vi "P3060_DMA读U32数据.vi"(8 "错误输入":errorcluster caption="错误输入（无错误）", 9 "数据长度":u32, 10 "偏移地址":u32, 11 "句柄输入":i32) -> (0 "错误输出":errorcluster, 1 "读I64数据":u32[](array[numeric]), 2 "返回值":i32, 3 "句柄输出":i32)   [LabVIEW 2010]
doc: "发送异步通道数据"
uses:
  dll/P3060.dll
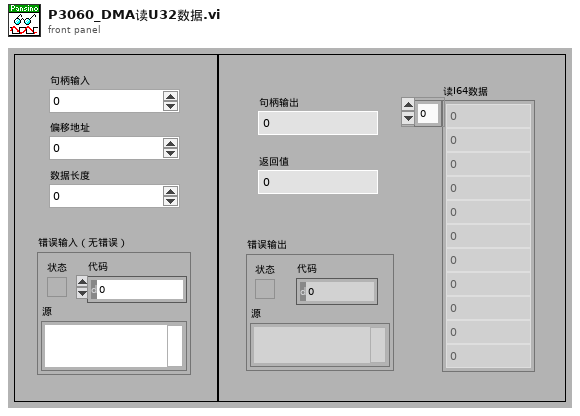
[diagram p1: front panel]
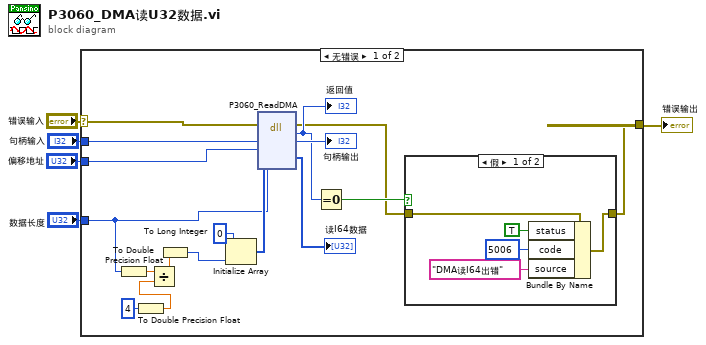
[diagram p0: block diagram]
diagram:
  n1 = case shown="无错误" "错误输入" {
    selector: "错误输入" -> [w22 w29]
    tunnel: [w16 w29] -> w3
    tunnel: "数据长度" -> [w6 _]
    tunnel: "句柄输入" -> [w20 _]
    tunnel: "偏移地址" -> [w15 _]
    frame No Error {
      n2 = To Double Precision Float(number=w6) -> (double precision float=w11:dbl)
      n3 = To Double Precision Float(number=u32 4 ("y")) -> (double precision float=w9:dbl)
      n4 = Divide(x=w11, y=w9) -> (x/y=w10:dbl)
      n5 = To Long Integer(number=w10) -> (32bit integer=w7:i32)
      n6 = Initialize Array(u32 0, w7) -> (w13:u32[])
      n7 = dll-call lib="D:/driver/trunk/Drivers/P3060/P3060API/P3060APILV/Labview/P3060/_SubVI/dll/P3060.dll" fn="P3060_ReadDMA"(error in=w22, "hDev"=w20, "Offset"=w15, "pBuffer"=w13, "lengthToWrite"=w6) -> (error out=w17:errorcluster, "return"=w19:i32, "hDev"=→"句柄输出":i32, "pBuffer"=→"读I64数据":u32[])  [unwired: 4 in, 1 out]
      "返回值" <- w19
      n8 = Equal To 0?(x=w19) -> (x = 0?=w18:bool)
      n9 = case shown="假" w18 {
        tunnel: [w26 w28] -> w16
        tunnel: w17 -> [w27 w28]
        frame False {
          n10 = Bundle By Name(cluster=w27, "status"=TRUE, "code"=5006, "source"="DMA读I64出错") -> (w26:errorcluster)
        }
        frame True {
        }
      }
    }
    frame Error {
    }
  }
  "错误输出" <- w3
